vi "Get IV and Ic distribution.vi"() -> ()   [LabVIEW 2017]
uses:
  <vilib>/LabVIEW Targets/FPGA/cRIO/shared/nicrio_ModuleControls/nicrio_cRIO-9775_RecordDataRates4ChansRing.ctl
  <resource>/objmgr/ni.dex.rc
  <vilib>/Analysis/NI_AALBase.lvlib
panel:
  out "Time to Init ms":u32
  out "Start time ms":u32
  in  "Wire resistance":dbl=1200.0
  in  "Read point":i32=1
  out "Done":bool=TRUE
  out "Array":dbl[](array[numeric])
  out "Histogram Graph":T1(graph)={"X Values"=[3.3134326171875, 3.3172509765625, 3.3210693359374996, 3.3248876953124995, 3.3287060546874994, 3.332524414062499, 3.336342773437499, 3.340161132812499, 3.343979492187499, 3.3477978515624986, 3.3516162109374985, 3.3554345703124984, 3.3592529296874982, 3.363071289062498, 3.366889648437498, 3.370708007812498, 3.3745263671874977, 3.3783447265624975, 3.3821630859374974, 3.3859814453124972, 3.389799804687497, 3.393618164062497, 3.397436523437497, 3.4012548828124967, 3.4050732421874965, 3.4088916015624964, 3.4127099609374962, 3.416528320312496, 3.420346679687496, 3.424165039062496, 3.4279833984374957, 3.4318017578124955, 3.4356201171874954, 3.4394384765624952, 3.443256835937495, 3.447075195312495, 3.450893554687495, 3.4547119140624947, 3.4585302734374945, 3.4623486328124944, 3.4661669921874942, 3.469985351562494, 3.473803710937494, 3.477622070312494, 3.4814404296874937, 3.4852587890624935, 3.4890771484374934, 3.4928955078124932, 3.496713867187493, 3.500532226562493, 3.504350585937493, 3.5081689453124927, 3.5119873046874925, 3.5158056640624924, 3.5196240234374923, 3.523442382812492, 3.527260742187492, 3.531079101562492, 3.5348974609374917, 3.5387158203124915, 3.5425341796874914, 3.5463525390624913, 3.550170898437491, 3.553989257812491, 3.557807617187491, 3.5616259765624907, 3.5654443359374905, 3.5692626953124904, 3.5730810546874903, 3.57689941406249, 3.58071777343749, 3.58453613281249, 3.5883544921874897, 3.5921728515624896, 3.5959912109374894, 3.5998095703124893, 3.603627929687489, 3.607446289062489, 3.611264648437489, 3.6150830078124887, 3.6189013671874886, 3.6227197265624884, 3.6265380859374883, 3.630356445312488, 3.634174804687488, 3.637993164062488, 3.6418115234374877, 3.6456298828124876, 3.6494482421874874, 3.6532666015624873, 3.657084960937487, 3.660903320312487, 3.664721679687487, 3.6685400390624867, 3.6723583984374866, 3.6761767578124864, 3.6799951171874863, 3.683813476562486, 3.687631835937486, 3.691450195312486], "Histogram: h(x)"=[1, 0, 0, 0, 0, 0, 0, 0, 0, 0, 0, 2, 1, 1, 0, 1, 0, 0, 1, 2, 1, 3, 0, 6, 4, 7, 10, 17, 12, 18, 19, 29, 31, 21, 42, 63, 53, 34, 61, 57, 79, 76, 106, 126, 134, 180, 77, 209, 227, 103, 268, 243, 246, 258, 208, 258, 334, 356, 209, 350, 364, 328, 188, 369, 359, 325, 236, 334, 278, 280, 266, 169, 251, 246, 141, 183, 188, 158, 124, 69, 117, 93, 90, 64, 55, 40, 31, 17, 22, 25, 15, 7, 4, 5, 4, 3, 4, 2, 1, 1]}
  in  "Ic parameters":T3={"Records Num"=10000, "AI Trigger Configuration"={"Trigger Slope"=enum."Positive", "Trigger Level"=0.550048828125, "Hystesis Value"=0.10009765625, "AI Channel"=0}, "Record PreTrigger Samples"=1, "Record Samples"=16, "Ic Cut off or curve"=TRUE, "Gate wait time us"=150, "Record Data Rate"=1} {"Record Data Rate" items=["20.000 MS/s (NI 9775)"=1, "10.00 MS/s (NI 9775)"=2, "6.667 MS/s (NI 9775)"=3, "5.000 MS/s (NI 9775)"=4, "2.500 MS/s (NI 9775)"=8, "1.667 MS/s (NI 9775)"=12, "1.250 MS/s (NI 9775)"=16, "1.000 MS/s (NI 9775)"=20, "833.333 KS/s (NI 9775)"=24, "714.286 KS/s (NI 9775)"=28, "625.000 KS/s (NI 9775)"=32, "555.556 KS/s (NI 9775)"=36, "500.000 KS/s (NI 9775)"=40, "454.545 KS/s (NI 9775)"=44, "416.667 KS/s (NI 9775)"=48, "384.615 KS/s (NI 9775)"=52, "357.143 KS/s (NI 9775)"=56, "333.333 KS/s (NI 9775)"=60, "312.500 KS/s (NI 9775)"=64, "294.118 KS/s (NI 9775)"=68, "277.778 KS/s (NI 9775)"=72, "263.158 KS/s (NI 9775)"=76, "250.000 KS/s (NI 9775)"=80, "238.095 KS/s (NI 9775)"=84, "227.273 KS/s (NI 9775)"=88, "217.391 KS/s (NI 9775)"=92, "208.333 KS/s (NI 9775)"=96, "200.000 KS/s (NI 9775)"=100, "192.308 KS/s (NI 9775)"=104, "185.185 KS/s (NI 9775)"=108, "178.571 KS/s (NI 9775)"=112, "172.414 KS/s (NI 9775)"=116, "166.667 KS/s (NI 9775)"=120, "161.290 KS/s (NI 9775)"=124, "156.250 KS/s (NI 9775)"=128, "151.515 KS/s (NI 9775)"=132, "147.059 KS/s (NI 9775)"=136, "142.857 KS/s (NI 9775)"=140, "138.889 KS/s (NI 9775)"=144, "135.135 KS/s (NI 9775)"=148, "131.579 KS/s (NI 9775)"=152, "128.205 KS/s (NI 9775)"=156, "125.000 KS/s (NI 9775)"=160, "121.951 KS/s (NI 9775)"=164, "119.048 KS/s (NI 9775)"=168, "116.279 KS/s (NI 9775)"=172, "113.636 KS/s (NI 9775)"=176, "111.111 KS/s (NI 9775)"=180, "108.696 KS/s (NI 9775)"=184, "106.383 KS/s (NI 9775)"=188, "104.167 KS/s (NI 9775)"=192, "102.041 KS/s (NI 9775)"=196, "100.000 KS/s (NI 9775)"=200, "50.000 KS/s (NI 9775)"=400, "33.333 KS/s (NI 9775)"=600, "25.000 KS/s (NI 9775)"=800, "20.000 KS/s (NI 9775)"=1000, "16.667 KS/s (NI 9775)"=1200, "14.286 KS/s (NI 9775)"=1400, "12.500 KS/s (NI 9775)"=1600, "11.111 KS/s (NI 9775)"=1800, "10.000 KS/s (NI 9775)"=2000, "9.091 KS/s (NI 9775)"=2200, "8.333 KS/s (NI 9775)"=2400, "7.692 KS/s (NI 9775)"=2600, "7.143 KS/s (NI 9775)"=2800, "6.667 KS/s (NI 9775)"=3000, "6.250 KS/s (NI 9775)"=3200, "5.882 KS/s (NI 9775)"=3400, "5.556 KS/s (NI 9775)"=3600, "5.000 KS/s (NI 9775)"=4000, "4.762 KS/s (NI 9775)"=4200, "4.545 KS/s (NI 9775)"=4400, "4.348 KS/s (NI 9775)"=4600, "4.167 KS/s (NI 9775)"=4800, "4.000 KS/s (NI 9775)"=5000, "3.846 KS/s (NI 9775)"=5200, "3.571 KS/s (NI 9775)"=5600, "3.333 KS/s (NI 9775)"=6000, "3.125 KS/s (NI 9775)"=6400, "2.941 KS/s (NI 9775)"=6800, "2.778 KS/s (NI 9775)"=7200, "2.632 KS/s (NI 9775)"=7600, "2.500 KS/s (NI 9775)"=8000, "2.381 KS/s (NI 9775)"=8400, "2.273 KS/s (NI 9775)"=8800, "2.174 KS/s (NI 9775)"=9200, "2.083 KS/s (NI 9775)"=9600, "2.000 KS/s (NI 9775)"=10000, "1.923 KS/s (NI 9775)"=10400, "1.852 KS/s (NI 9775)"=10800, "1.786 KS/s (NI 9775)"=11200, "1.724 KS/s (NI 9775)"=11600, "1.667 KS/s (NI 9775)"=12000, "1.613 KS/s (NI 9775)"=12400, "1.563 KS/s (NI 9775)"=12800, "1.515 KS/s (NI 9775)"=13200, "1.471 KS/s (NI 9775)"=13600, "1.429 KS/s (NI 9775)"=14000, "1.389 KS/s (NI 9775)"=14400, "1.351 KS/s (NI 9775)"=14800, "1.316 KS/s (NI 9775)"=15200, "1.282 KS/s (NI 9775)"=15600, "1.250 KS/s (NI 9775)"=16000, "1.220 KS/s (NI 9775)"=16400, "1.190 KS/s (NI 9775)"=16800, "1.163 KS/s (NI 9775)"=17200, "1.136 KS/s (NI 9775)"=17600, "1.111 KS/s (NI 9775)"=18000, "1.087 KS/s (NI 9775)"=18400, "1.064 KS/s (NI 9775)"=18800, "1.042 KS/s (NI 9775)"=19200, "1.020 KS/s (NI 9775)"=19600, "1.000 KS/s (NI 9775)"=20000, "0.980 KS/s (NI 9775)"=20400, "0.962 KS/s (NI 9775)"=20800, "0.943 KS/s (NI 9775)"=21200, "0.926 KS/s (NI 9775)"=21600, "0.909 KS/s (NI 9775)"=22000, "0.893 KS/s (NI 9775)"=22400, "0.877 KS/s (NI 9775)"=22800, "0.862 KS/s (NI 9775)"=23200, "0.847 KS/s (NI 9775)"=23600, "0.833 KS/s (NI 9775)"=24000, "0.820 KS/s (NI 9775)"=24400, "0.806 KS/s (NI 9775)"=24800, "0.794 KS/s (NI 9775)"=25200, "0.781 KS/s (NI 9775)"=25600, "0.694 KS/s (NI 9775)"=28800, "0.625 KS/s (NI 9775)"=32000, "0.568 KS/s (NI 9775)"=35200, "0.521 KS/s (NI 9775)"=38400, "0.446 KS/s (NI 9775)"=44800, "0.391 KS/s (NI 9775)"=51200, "0.347 KS/s (NI 9775)"=57600, "0.313 KS/s (NI 9775)"=64000]}
  in  "IV parameters":T3={"Records Num"=1, "AI Trigger Configuration"={"Trigger Slope"=enum."Positive", "Trigger Level"=0.10009765625, "Hystesis Value"=0.094970703125, "AI Channel"=0}, "Record PreTrigger Samples"=1, "Record Samples"=5000, "Ic Cut off or curve"=FALSE, "Gate wait time us"=150, "Record Data Rate"=200} {"Record Data Rate" items=["20.000 MS/s (NI 9775)"=1, "10.00 MS/s (NI 9775)"=2, "6.667 MS/s (NI 9775)"=3, "5.000 MS/s (NI 9775)"=4, "2.500 MS/s (NI 9775)"=8, "1.667 MS/s (NI 9775)"=12, "1.250 MS/s (NI 9775)"=16, "1.000 MS/s (NI 9775)"=20, "833.333 KS/s (NI 9775)"=24, "714.286 KS/s (NI 9775)"=28, "625.000 KS/s (NI 9775)"=32, "555.556 KS/s (NI 9775)"=36, "500.000 KS/s (NI 9775)"=40, "454.545 KS/s (NI 9775)"=44, "416.667 KS/s (NI 9775)"=48, "384.615 KS/s (NI 9775)"=52, "357.143 KS/s (NI 9775)"=56, "333.333 KS/s (NI 9775)"=60, "312.500 KS/s (NI 9775)"=64, "294.118 KS/s (NI 9775)"=68, "277.778 KS/s (NI 9775)"=72, "263.158 KS/s (NI 9775)"=76, "250.000 KS/s (NI 9775)"=80, "238.095 KS/s (NI 9775)"=84, "227.273 KS/s (NI 9775)"=88, "217.391 KS/s (NI 9775)"=92, "208.333 KS/s (NI 9775)"=96, "200.000 KS/s (NI 9775)"=100, "192.308 KS/s (NI 9775)"=104, "185.185 KS/s (NI 9775)"=108, "178.571 KS/s (NI 9775)"=112, "172.414 KS/s (NI 9775)"=116, "166.667 KS/s (NI 9775)"=120, "161.290 KS/s (NI 9775)"=124, "156.250 KS/s (NI 9775)"=128, "151.515 KS/s (NI 9775)"=132, "147.059 KS/s (NI 9775)"=136, "142.857 KS/s (NI 9775)"=140, "138.889 KS/s (NI 9775)"=144, "135.135 KS/s (NI 9775)"=148, "131.579 KS/s (NI 9775)"=152, "128.205 KS/s (NI 9775)"=156, "125.000 KS/s (NI 9775)"=160, "121.951 KS/s (NI 9775)"=164, "119.048 KS/s (NI 9775)"=168, "116.279 KS/s (NI 9775)"=172, "113.636 KS/s (NI 9775)"=176, "111.111 KS/s (NI 9775)"=180, "108.696 KS/s (NI 9775)"=184, "106.383 KS/s (NI 9775)"=188, "104.167 KS/s (NI 9775)"=192, "102.041 KS/s (NI 9775)"=196, "100.000 KS/s (NI 9775)"=200, "50.000 KS/s (NI 9775)"=400, "33.333 KS/s (NI 9775)"=600, "25.000 KS/s (NI 9775)"=800, "20.000 KS/s (NI 9775)"=1000, "16.667 KS/s (NI 9775)"=1200, "14.286 KS/s (NI 9775)"=1400, "12.500 KS/s (NI 9775)"=1600, "11.111 KS/s (NI 9775)"=1800, "10.000 KS/s (NI 9775)"=2000, "9.091 KS/s (NI 9775)"=2200, "8.333 KS/s (NI 9775)"=2400, "7.692 KS/s (NI 9775)"=2600, "7.143 KS/s (NI 9775)"=2800, "6.667 KS/s (NI 9775)"=3000, "6.250 KS/s (NI 9775)"=3200, "5.882 KS/s (NI 9775)"=3400, "5.556 KS/s (NI 9775)"=3600, "5.000 KS/s (NI 9775)"=4000, "4.762 KS/s (NI 9775)"=4200, "4.545 KS/s (NI 9775)"=4400, "4.348 KS/s (NI 9775)"=4600, "4.167 KS/s (NI 9775)"=4800, "4.000 KS/s (NI 9775)"=5000, "3.846 KS/s (NI 9775)"=5200, "3.571 KS/s (NI 9775)"=5600, "3.333 KS/s (NI 9775)"=6000, "3.125 KS/s (NI 9775)"=6400, "2.941 KS/s (NI 9775)"=6800, "2.778 KS/s (NI 9775)"=7200, "2.632 KS/s (NI 9775)"=7600, "2.500 KS/s (NI 9775)"=8000, "2.381 KS/s (NI 9775)"=8400, "2.273 KS/s (NI 9775)"=8800, "2.174 KS/s (NI 9775)"=9200, "2.083 KS/s (NI 9775)"=9600, "2.000 KS/s (NI 9775)"=10000, "1.923 KS/s (NI 9775)"=10400, "1.852 KS/s (NI 9775)"=10800, "1.786 KS/s (NI 9775)"=11200, "1.724 KS/s (NI 9775)"=11600, "1.667 KS/s (NI 9775)"=12000, "1.613 KS/s (NI 9775)"=12400, "1.563 KS/s (NI 9775)"=12800, "1.515 KS/s (NI 9775)"=13200, "1.471 KS/s (NI 9775)"=13600, "1.429 KS/s (NI 9775)"=14000, "1.389 KS/s (NI 9775)"=14400, "1.351 KS/s (NI 9775)"=14800, "1.316 KS/s (NI 9775)"=15200, "1.282 KS/s (NI 9775)"=15600, "1.250 KS/s (NI 9775)"=16000, "1.220 KS/s (NI 9775)"=16400, "1.190 KS/s (NI 9775)"=16800, "1.163 KS/s (NI 9775)"=17200, "1.136 KS/s (NI 9775)"=17600, "1.111 KS/s (NI 9775)"=18000, "1.087 KS/s (NI 9775)"=18400, "1.064 KS/s (NI 9775)"=18800, "1.042 KS/s (NI 9775)"=19200, "1.020 KS/s (NI 9775)"=19600, "1.000 KS/s (NI 9775)"=20000, "0.980 KS/s (NI 9775)"=20400, "0.962 KS/s (NI 9775)"=20800, "0.943 KS/s (NI 9775)"=21200, "0.926 KS/s (NI 9775)"=21600, "0.909 KS/s (NI 9775)"=22000, "0.893 KS/s (NI 9775)"=22400, "0.877 KS/s (NI 9775)"=22800, "0.862 KS/s (NI 9775)"=23200, "0.847 KS/s (NI 9775)"=23600, "0.833 KS/s (NI 9775)"=24000, "0.820 KS/s (NI 9775)"=24400, "0.806 KS/s (NI 9775)"=24800, "0.794 KS/s (NI 9775)"=25200, "0.781 KS/s (NI 9775)"=25600, "0.694 KS/s (NI 9775)"=28800, "0.625 KS/s (NI 9775)"=32000, "0.568 KS/s (NI 9775)"=35200, "0.521 KS/s (NI 9775)"=38400, "0.446 KS/s (NI 9775)"=44800, "0.391 KS/s (NI 9775)"=51200, "0.347 KS/s (NI 9775)"=57600, "0.313 KS/s (NI 9775)"=64000]}
  out "XY Graph":cluster{"Y":dbl[], "Y":dbl[]}[](graph)
  in  "Data buffer size":i32=1000
  in  "stop":bool
  out "error out":errorcluster={"status"=FALSE, "code"=180121605, "source"="Shared Variable in Get IV and Ic distribution.vi<APPEND>\nThis error or warning occurred while writing the following Shared Variable:\n\\\\NI-cRIO-9063-01bc8cc6\\network varibles\\RT Stop\n\\\\172.22.11.2\\network varibles\\RT Stop"}
  in  "cRIO IP":string="//172.22.11.2"
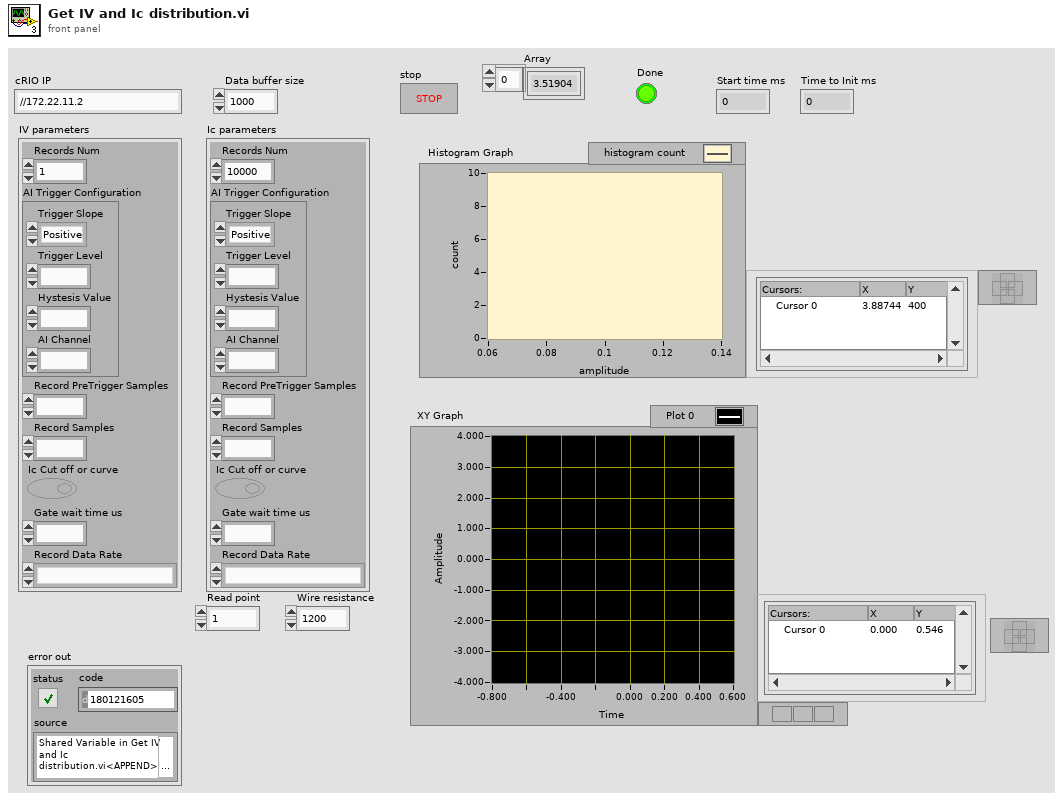
[diagram p1: front panel]
types:
  T1 = cluster{"X Values":dbl[], "Histogram: h(x)":i32[]}
  T2 = typedef "nicrio_cRIO-9775_RecordDataRates4ChansRing.ctl" = u16
  T3 = cluster{"Records Num":i32, "AI Trigger Configuration":cluster{"Trigger Slope":enum8{"Positive", "Negative"}, "Trigger Level":fxp<+/-,17,5>, "Hystesis Value":fxp<+,16,4>, "AI Channel":u8}, "Record PreTrigger Samples":u32, "Record Samples":u32, "Ic Cut off or curve":bool, "Gate wait time us":u32, "Record Data Rate":T2}
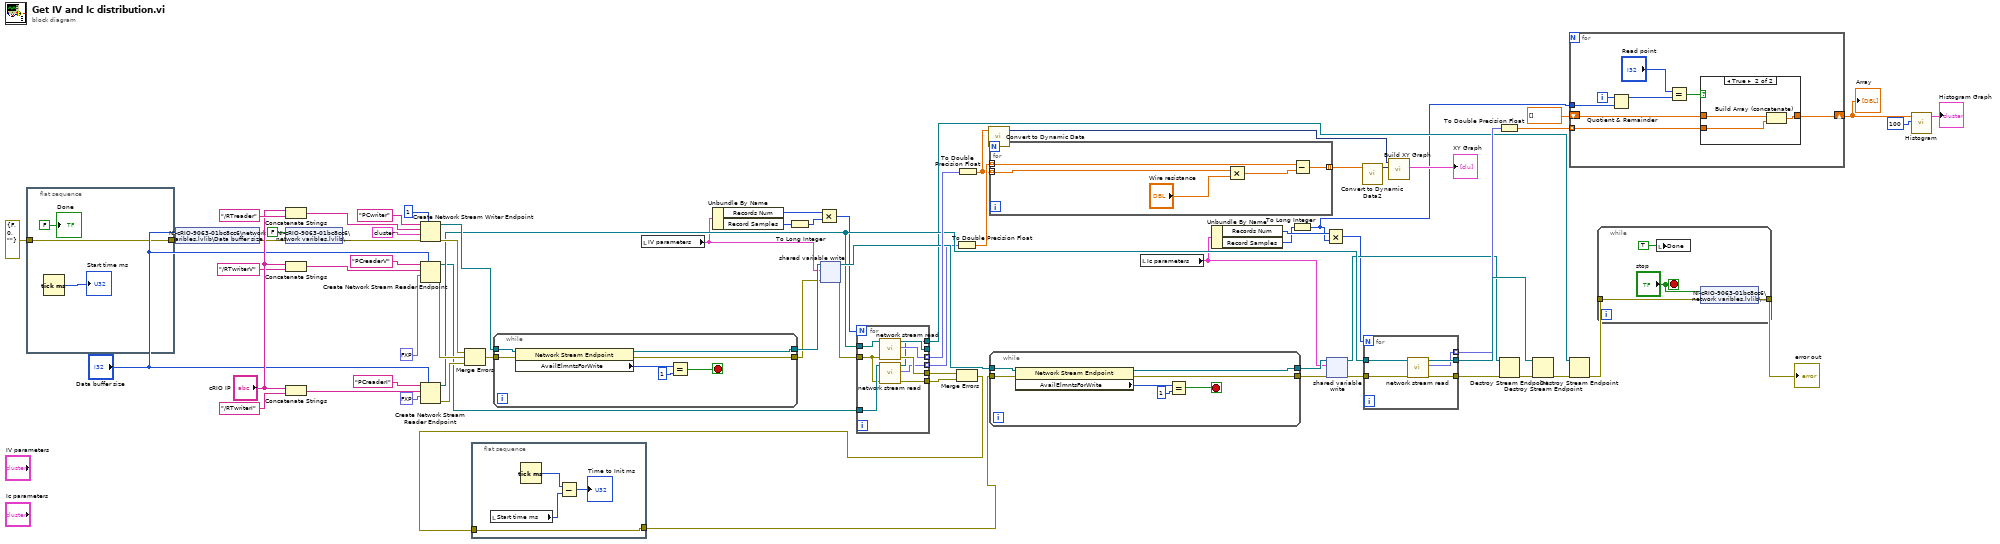
[diagram p0: block diagram]
diagram:
  n1 = flat-sequence {
    tunnel: [w72] -> w8
    tunnel: errorcluster {"status"=FALSE, "code"=0, "source"=""} ("error in (no error)") -> [w72]
    frame #0 {
      n2 = Tick Count (ms)() -> (millisecond timer value=→"Start time ms":u32)
      "Done" <- FALSE ("Done")
    }
  }
  n3 = shared-variable "NI-cRIO-9063-01bc8cc6\\network varibles.lvlib\\Data buffer size"("Data buffer size", error in=w8) -> (error out=w47:errorcluster)
  n4 = shared-variable "NI-cRIO-9063-01bc8cc6\\network varibles.lvlib\\RT Stop"(FALSE ("RT Stop"), error in=w47) -> (error out=w55:errorcluster)
  n5 = Concatenate Strings("cRIO IP", "/RTreader" ("string")) -> (w65:string)
  n6 = Concatenate Strings("cRIO IP", "/RTwriterV" ("string")) -> (w57:string)
  n7 = Concatenate Strings("cRIO IP", "/RTwriterI" ("string")) -> (w49:string)
  n8 = Create Network Stream Writer Endpoint(7:1 ("writer buffer size"), 8:w55, 9:T3 {"Records Num"=0, "AI Trigger Configuration"={"Trigger Slope"=enum."Positive", "Trigger Level"=0.0, "Hystesis Value"=0.0, "AI Channel"=0}, "Record PreTrigger Samples"=0, "Record Samples"=0, "Ic Cut off or curve"=FALSE, "Gate wait time us"=0, "Record Data Rate"=1} ("Parameters 4"), 10:w65, 11:"PCwriter" ("writer name")) -> (0:w63:errorcluster, 3:w62:refnum<k21>)  [unwired: 2 in]
  n9 = Create Network Stream Reader Endpoint(7:"Data buffer size", 9:fxp<+/-,17,5> 0.0, 10:w57, 11:"PCreaderV" ("reader name")) -> (0:w54:errorcluster, 3:w22:refnum<k21>)  [unwired: 3 in]
  n10 = Create Network Stream Reader Endpoint(7:"Data buffer size", 9:fxp<+/-,17,5> 0.0, 10:w49, 11:"PCreaderI" ("reader name")) -> (0:w46:errorcluster, 3:w39:refnum<k21>)  [unwired: 3 in]
  n11 = Merge Errors(w63, w54, w46) -> (w61:errorcluster)
  n12 = flat-sequence {
    tunnel: w2 -> [w74]
    tunnel: [w74] -> w1
    frame #0 {
      n13 = local read "Start time ms"() -> (w76:u32)
      n14 = Tick Count (ms)() -> (millisecond timer value=w77:u32)
      n15 = Subtract(x=w77, y=w76) -> (x-y=→"Time to Init ms":u32)
    }
  }
  n16 = while {
    tunnel: w62 -> [w84]
    tunnel: w61 -> [w83]
    tunnel: [w79] -> w67
    tunnel: [w78] -> w4
    stop <- w80 stop-if-true
    n17 = property class="Network Stream Endpoint"(reference=w84, error in=w83) -> (reference out=w79:refnum<k21>, error out=w78:errorcluster, "AvailElmntsForWrite"=w82:i32)
    n18 = Equal?(x=w82, y=1) -> (x = y?=w80:bool)
  }
  n19 = local read "IV parameters"() -> (w27:T3)
  n20 = Unbundle By Name(w27) -> ("Records Num"=w26:i32, "Record Samples"=w25:u32)
  n21 = To Long Integer(number=w25) -> (32bit integer=w24:i32)
  n22 = Multiply(x=w26, y=w24) -> (x*y=w23:i32)
  n23 = shared-variable-write(w67, w4, w27) -> (w42:refnum<k21>, w3:errorcluster)  [unwired: 1 in, 1 out]
  n24 = for {
    N: w23 -> [_]
    tunnel: w39 -> [w93]
    tunnel: w3 -> [w86]
    tunnel: [w92] -> w45 mode=indexing
    tunnel: [w91] -> _
    tunnel: [w90] -> w18
    tunnel: w22 -> [w89]
    tunnel: [w88] -> w21
    tunnel: [w87] -> w19 mode=indexing
    tunnel: [w85] -> w17
    n25 = call "network stream read.vi"("error in (no error)"=w86, "endpoint in"=w93) -> ("error out"=w90:errorcluster, "Data"=w92:fxp<+/-,17,5>, "endpoint out"=w91:refnum<k21>)  [unwired: 7 in]
    n26 = call "network stream read.vi"("error in (no error)"=w86, "endpoint in"=w89) -> ("error out"=w85:errorcluster, "Data"=w87:fxp<+/-,17,5>, "endpoint out"=w88:refnum<k21>)  [unwired: 7 in]
  }
  n27 = To Double Precision Float(number=w19) -> (double precision float=w7:dbl[])
  n28 = Merge Errors(w18, w17) -> (w2:errorcluster)
  n29 = To Double Precision Float(number=w45) -> (double precision float=w6:dbl[])
  n30 = call "Convert to Dynamic Data"("Array"=w6) -> ("Dynamic Data Type"=w33:dynamicdata)  [unwired: 3 in]
  n31 = for {
    tunnel: w7 -> [w98] mode=indexing
    tunnel: w6 -> [w96] mode=indexing
    tunnel: [w94] -> w5 mode=indexing
    n32 = Multiply(x=w96, y="Wire resistance") -> (x*y=w95:dbl)
    n33 = Subtract(x=w98, y=w95) -> (x-y=w94:dbl)
  }
  n34 = while {
    tunnel: w42 -> [w103]
    tunnel: w1 -> [w102]
    tunnel: [w100] -> w41
    tunnel: [w99] -> w40
    stop <- w101 stop-if-true
    n35 = property class="Network Stream Endpoint"(reference=w103, error in=w102) -> (reference out=w100:refnum<k21>, error out=w99:errorcluster, "AvailElmntsForWrite"=w105:i32)
    n36 = Equal?(x=w105, y=1) -> (x = y?=w101:bool)
  }
  n37 = local read "Ic parameters"() -> (w31:T3)
  n38 = Unbundle By Name(w31) -> ("Records Num"=w30:i32, "Record Samples"=w29:u32)
  n39 = To Long Integer(number=w29) -> (32bit integer=w12:i32)
  n40 = Multiply(x=w30, y=w12) -> (x*y=w28:i32)
  n41 = shared-variable-write(w41, w40, w31) -> (w34:refnum<k21>, w38:errorcluster)  [unwired: 1 in, 1 out]
  n42 = call "Convert to Dynamic Data2"("Array"=w5) -> ("Dynamic Data Type"=w32:dynamicdata)  [unwired: 3 in]
  n43 = for {
    N: w28 -> [_]
    tunnel: w39 -> [w110]
    tunnel: w38 -> [w109]
    tunnel: [w108] -> w20
    tunnel: [w107] -> w37
    tunnel: [w106] -> w35 mode=indexing
    n44 = call "network stream read.vi"("error in (no error)"=w109, "endpoint in"=w110) -> ("error out"=w108:errorcluster, "Data"=w106:fxp<+/-,17,5>, "endpoint out"=w107:refnum<k21>)  [unwired: 7 in]
  }
  n45 = call "Build XY Graph"("Y Input"=w32, "X Input"=w33) -> ("XY Graph"=→"XY Graph":cluster{"X":dbl[], "Y":dbl[]}[])  [unwired: 8 in, 1 out]
  n46 = To Double Precision Float(number=w35) -> (double precision float=w13:dbl[])
  n47 = Destroy Stream Endpoint(8:w20, 11:w34) -> (0:w53:errorcluster)
  n48 = Destroy Stream Endpoint(8:w53, 11:w37) -> (0:w44:errorcluster)
  n49 = for {
    tunnel: w13 -> [w112] mode=indexing
    tunnel: w12 -> [w118]
    shift-right: [w114] -> w10
    shift-left: dbl[] [] -> [w113]
    i -> [w117]
    n50 = Quotient & Remainder(x=w117, y=w118) -> (x-y*floor(x/y)=w116:i32)  [unwired: 1 out]
    n51 = Equal?(x="Read point", y=w116) -> (x = y?=w111:bool)
    n52 = case shown="True" w111 {
      tunnel: [w119 w122] -> w114
      tunnel: w113 -> [w119 w121]
      tunnel: w112 -> [_ w120]
      frame False {
      }
      frame True {
        n53 = Build Array (concatenate)(w121, w120) -> (w122:dbl[])
      }
    }
  }
  "Array" <- w10
  n54 = Destroy Stream Endpoint(8:w44, 11:w21) -> (0:w43:errorcluster)
  n55 = while {
    tunnel: w43 -> [w125]
    tunnel: [w124] -> w52
    stop <- "stop" stop-if-true
    n56 = local write "Done"(TRUE ("Done")) -> ()
    n57 = shared-variable "NI-cRIO-9063-01bc8cc6\\network varibles.lvlib\\RT Stop"("stop", error in=w125) -> (error out=w124:errorcluster)
  }
  "error out" <- w52
  n58 = call <vilib>:"Histogram.vi"("intervals"=100, "X"=w10) -> ("Histogram Graph"=→"Histogram Graph":T1)  [unwired: 6 in, 3 out]
